vi "Copy Value.vi"(10 "From":refnum<class "Type.lvclass">, 11 "ID in":refnum<class "ID.lvclass">) -> (2 "error out":errorcluster, 3 "ID out":refnum<class "ID.lvclass">)   [LabVIEW 2020, in "Conditu2.lvlib" / "Columns.lvlib" / "ID.lvclass"]
uses:
  ID.lvclass
  Type/Type.lvclass
  ID.lvclass/ID.ctl
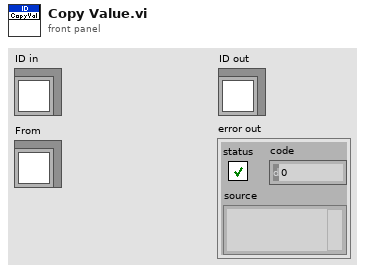
[diagram p1: front panel]
types:
  T1 = typedef "Conditu2.lvlib/Entity ID.ctl" = i64
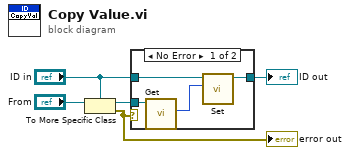
[diagram p0: block diagram]
diagram:
  n1 = To More Specific Class(target class="ID in", reference="From") -> (specific class reference=w5:refnum<class "ID.lvclass">, error out=w2:errorcluster)  [unwired: 1 in]
  "error out" <- w2
  n2 = case shown="No Error" w2 {
    tunnel: w5 -> [w9 _]
    tunnel: "ID in" -> [w7 w10]
    tunnel: [w6 w10] -> w1
    frame No Error {
      n3 = call "Get.vi"("ID in"=w9) -> ("Entity ID"=w8:T1)  [unwired: 10 in]
      n4 = call "Set.vi"("Entity ID"=w8, "ID in"=w7) -> ("ID out"=w6:refnum<class "ID.lvclass">)  [unwired: 9 in]
    }
    frame Error {
    }
  }
  "ID out" <- w1
